vi "Set-Exposure-time.vi"(7 "Camera":u32, 8 "error in (no error)":errorcluster, 10 "Acquis. params. ref. in":refnum<data-value>, 11 "PF_MV1-D1312-240 in":refnum<class "PF_MV1-D1312-240.lvclass">) -> (0 "error out":errorcluster, 1 "Exposure time":dbl caption="Exposure time [s]", 2 "Acquis. params. ref.":refnum<data-value>, 3 "PF_MV1-D1312-240 out":refnum<class "PF_MV1-D1312-240.lvclass">)   [LabVIEW 2013, in "CameraVision.lvlib" / "PF_MV1-D1312-240.lvclass"]
uses:
  PF_MV1-D1312-240.lvclass
  Main/Acquisition/CV-Acquisition.lvclass
  Camera.lvclass/Camera.ctl
  Main/Acquisition/CV-Acquisition.lvclass/CV-Acquisition.ctl
  Main/Acquisition/Read Exposure time camera 1.vi
  Main/Acquisition/Read Exposure time camera 2.vi
  <userlib>/Photonfocus Toolkit/_Public/SubVIs/pf_Set_Camera_Property_Float.vi
  <userlib>/Photonfocus Toolkit/Photonfocus_Toolkit.lvlib
  Camera.lvclass
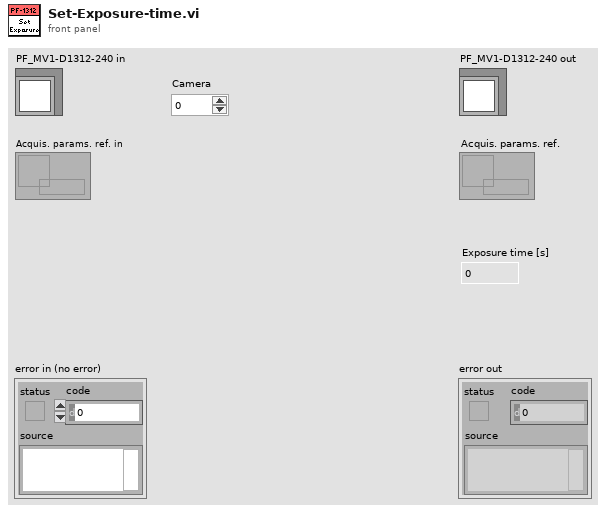
[diagram p1: front panel]
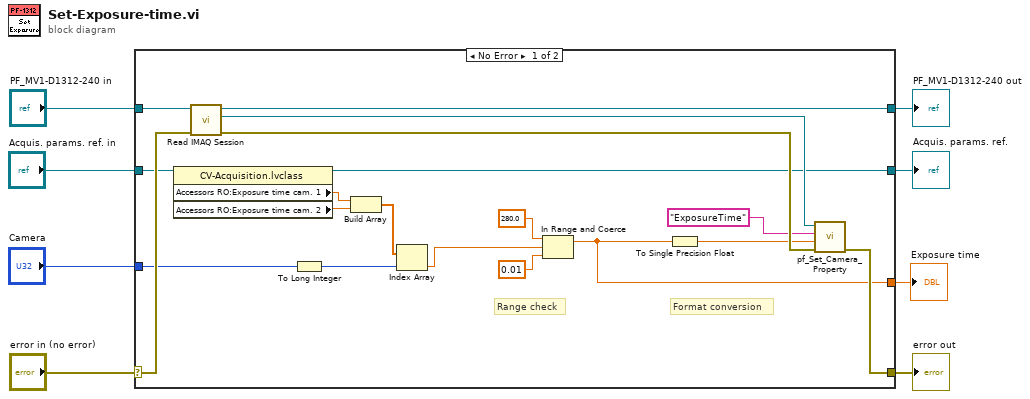
[diagram p0: block diagram]
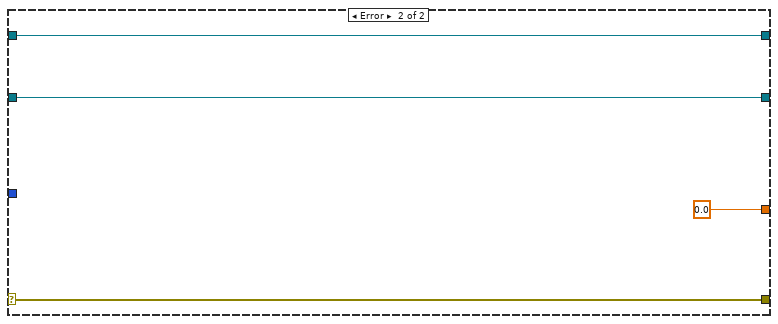
[diagram p2: hidden frame]
diagram:
  n1 = case shown="No Error" "error in (no error)" {
    selector: "error in (no error)" -> [w24 w31]
    tunnel: [w22 w31] -> w7
    tunnel: [w25 w30] -> w5
    tunnel: "PF_MV1-D1312-240 in" -> [w26 w30]
    tunnel: "Acquis. params. ref. in" -> [w17 w28]
    tunnel: [w11 0.0 ("upper limit")] -> w3
    tunnel: "Camera" -> [w13 _]
    tunnel: [w9 w28] -> w1
    frame No Error {
      # "Format conversion"
      # "Range check"
      n2 = property class="CV-Acquisition.lvclass"(reference=w17) -> (reference out=w9:refnum<data-value>, "Accessors RO:Exposure time cam. 1"=w16:dbl, "Accessors RO:Exposure time cam. 2"=w15:dbl)  [unwired: 1 in, 1 out]
      n3 = call "Read IMAQ Session.vi"("error in (no error)"=w24, "Camera in"=w26) -> ("error out"=w23:errorcluster, "IMAQ Session"=w27:refnum<k11>, "Camera out"=w25:refnum<class "PF_MV1-D1312-240.lvclass">)  [unwired: 7 in]
      n4 = To Long Integer(number=w13) -> (32bit integer=w12:i32)
      n5 = Build Array(w16, w15) -> (w14:dbl[])
      n6 = Index Array(array=w14, index=w12) -> (element=w10:dbl)
      n7 = In Range and Coerce(upper limit=280.0, x=w10, lower limit=0.01) -> (coerced(x)=w11:dbl)  [unwired: 1 out]
      n8 = To Single Precision Float(number=w11) -> (single precision float=w18:sgl)
      n9 = call-poly <userlib>:"pf_Set_Camera_Property.vi"("error in (no error)"=w23, "Property Value"=w18, "Property Name"="ExposureTime", "IMAQ Session in"=w27) -> ("error out"=w22:errorcluster)  [unwired: 5 in, 2 out]
    }
    frame Error {
    }
  }
  "error out" <- w7
  "PF_MV1-D1312-240 out" <- w5
  "Exposure time" <- w3
  "Acquis. params. ref." <- w1
